vi "CRYTree Global Manipulate.vi"(7 "sAction":string, 10 "sOption":string, 11 "Type In":enum16{"Curves", "Values", "Results", "WFM"}(ring)) -> (0 "WFM Tree":refnum<vi>, 1 "Results Tree":refnum<vi>, 2 "Values Tree":refnum<vi>, 3 "Tree/Curve Tree":refnum<vi>)   [LabVIEW 2013]
uses:
  Global/CRYCurve Library Global.vi
panel:
  in  "Curve Items":T1(array[cluster])
  in  "Value Items":T1(array[cluster])
  in  "Result Items":T1(array[cluster])
  in  "WFM Items":T1(array[cluster])
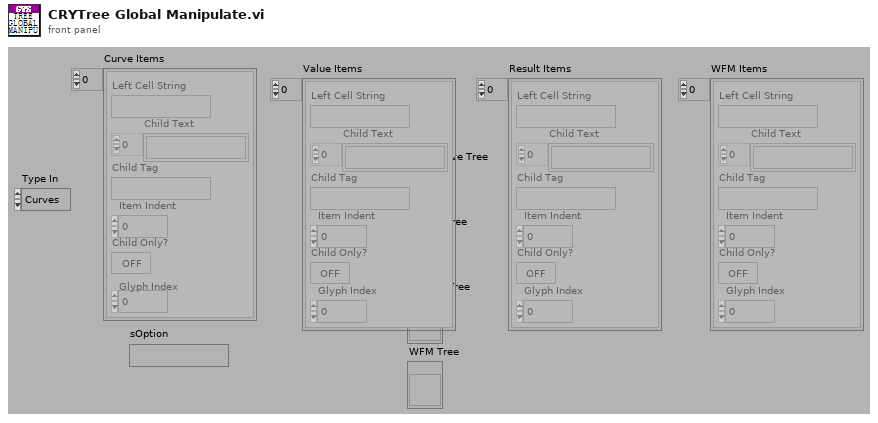
[diagram p1: front panel]
types:
  T1 = cluster{"Left Cell String":string, "Child Text":string[], "Child Tag":string, "Item Indent":i32, "Child Only?":bool, "Glyph Index":i32}[]
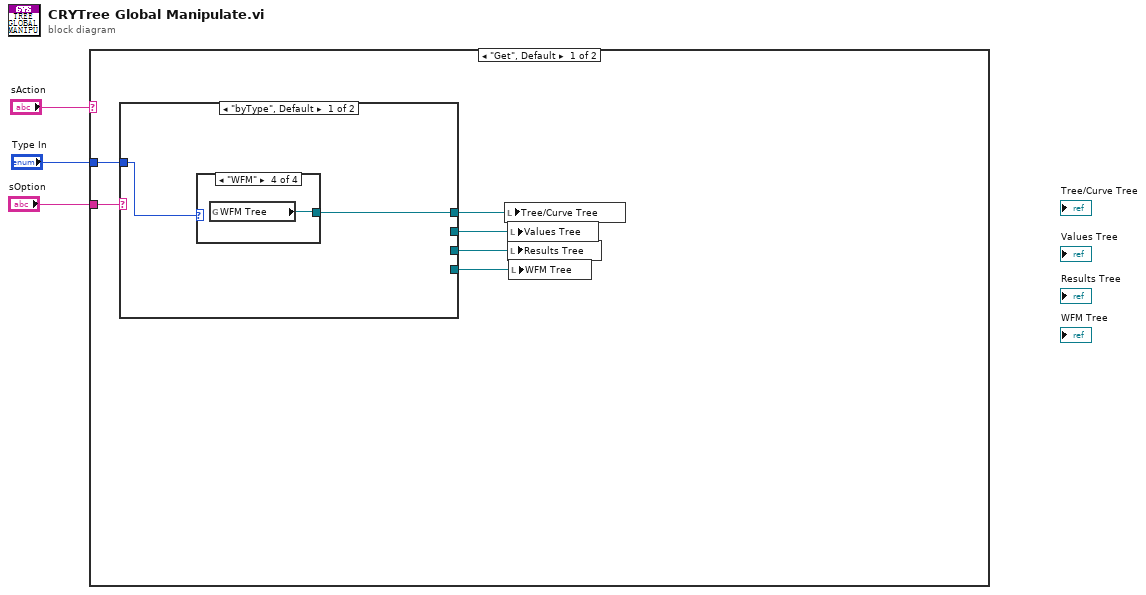
[diagram p0: block diagram]
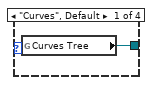
[diagram p2: hidden frame]
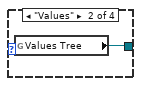
[diagram p3: hidden frame]
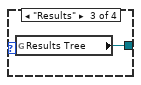
[diagram p4: hidden frame]
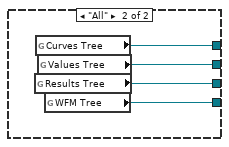
[diagram p5: hidden frame]
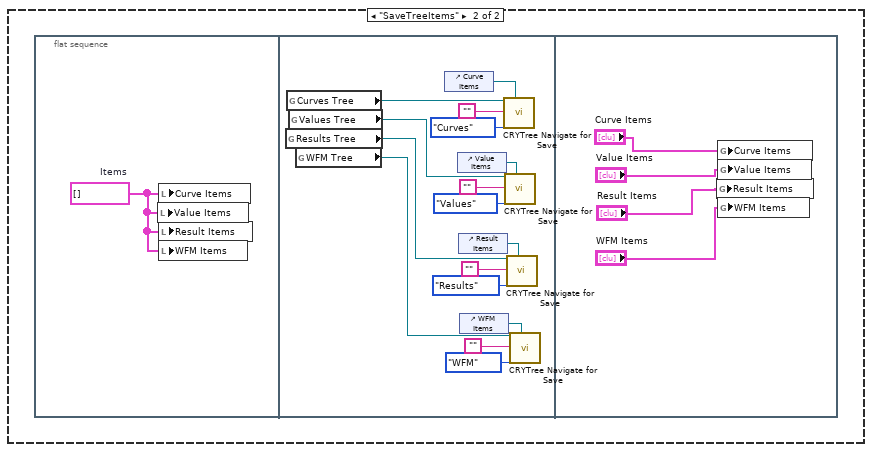
[diagram p6: hidden frame]
diagram:
  n1 = case shown="\"Get\", Default" "sAction" {
    tunnel: "sOption" -> [w9 _]
    tunnel: "Type In" -> [w8 _]
    frame "Get", Default {
      n2 = case shown="\"byType\", Default" w9 {
        tunnel: w8 -> [w11 _]
        tunnel: [w10 w19] -> w7
        tunnel: [_ w18] -> w6
        tunnel: [_ w17] -> w5
        tunnel: [_ w16] -> w4
        frame "byType", Default {
          n3 = case shown="\"WFM\"" w11 {
            tunnel: [w12 w13 w14 w15] -> w10
            frame "Curves", Default {
              n4 = global read "CRYCurve Library Global.vi" "Curves Tree"() -> (w12:refnum<vi>)
            }
            frame "Values" {
              n5 = global read "CRYCurve Library Global.vi" "Values Tree"() -> (w13:refnum<vi>)
            }
            frame "Results" {
              n6 = global read "CRYCurve Library Global.vi" "Results Tree"() -> (w14:refnum<vi>)
            }
            frame "WFM" {
              n7 = global read "CRYCurve Library Global.vi" "WFM Tree"() -> (w15:refnum<vi>)
            }
          }
        }
        frame "All" {
          n8 = global read "CRYCurve Library Global.vi" "Results Tree"() -> (w17:refnum<vi>)
          n9 = global read "CRYCurve Library Global.vi" "Curves Tree"() -> (w19:refnum<vi>)
          n10 = global read "CRYCurve Library Global.vi" "Values Tree"() -> (w18:refnum<vi>)
          n11 = global read "CRYCurve Library Global.vi" "WFM Tree"() -> (w16:refnum<vi>)
        }
      }
      n12 = local write "Tree/Curve Tree"(w7) -> ()
      n13 = local write "Values Tree"(w6) -> ()
      n14 = local write "Results Tree"(w5) -> ()
      n15 = local write "WFM Tree"(w4) -> ()
    }
    frame "SaveTreeItems" {
      n16 = flat-sequence {
        frame #0 {
          w20 = T1 []  # Items
          n17 = local write "Value Items"(w20) -> ()
          n18 = local write "Curve Items"(w20) -> ()
          n19 = local write "Result Items"(w20) -> ()
          n20 = local write "WFM Items"(w20) -> ()
        }
        frame #1 {
          n21 = global read "CRYCurve Library Global.vi" "Results Tree"() -> (w22:refnum<vi>)
          n22 = global read "CRYCurve Library Global.vi" "Curves Tree"() -> (w24:refnum<vi>)
          n23 = global read "CRYCurve Library Global.vi" "Values Tree"() -> (w23:refnum<vi>)
          n24 = global read "CRYCurve Library Global.vi" "WFM Tree"() -> (w21:refnum<vi>)
          n25 = control-ref of="Curve Items"() -> (w36:refnum<vi>)
          n26 = control-ref of="Value Items"() -> (w27:refnum<vi>)
          n27 = control-ref of="Result Items"() -> (w26:refnum<vi>)
          n28 = control-ref of="WFM Items"() -> (w25:refnum<vi>)
          n29 = call "CRYTree Navigate for Save.vi"("Items"=w36, "Type"=enum16{"Curves", "Values", "Results", "WFM"}."Curves", "Start Tag In"="", "Tree In"=w24) -> ()  [unwired: 7 in, 1 out]
          n30 = call "CRYTree Navigate for Save.vi"("Items"=w27, "Type"=enum16{"Curves", "Values", "Results", "WFM"}."Values", "Start Tag In"="", "Tree In"=w23) -> ()  [unwired: 7 in, 1 out]
          n31 = call "CRYTree Navigate for Save.vi"("Items"=w26, "Type"=enum16{"Curves", "Values", "Results", "WFM"}."Results", "Start Tag In"="", "Tree In"=w22) -> ()  [unwired: 7 in, 1 out]
          n32 = call "CRYTree Navigate for Save.vi"("Items"=w25, "Type"=enum16{"Curves", "Values", "Results", "WFM"}."WFM", "Start Tag In"="", "Tree In"=w21) -> ()  [unwired: 7 in, 1 out]
        }
        frame #2 {
          n33 = global write "CRYCurve Library Global.vi" "Result Items"("Result Items") -> ()
          n34 = global write "CRYCurve Library Global.vi" "Curve Items"("Curve Items") -> ()
          n35 = global write "CRYCurve Library Global.vi" "Value Items"("Value Items") -> ()
          n36 = global write "CRYCurve Library Global.vi" "WFM Items"("WFM Items") -> ()
        }
      }
    }
  }
